vi "add_string_to_array_unique.vi"(8 "error in (no error)":errorcluster, 10 "strings to add":string[](array[string])=["subcomponent_cluster.ctl"], 11 "array in":string[](array[string])) -> (0 "error out":errorcluster, 3 "array out":string[](array[string]))   [LabVIEW 2010]
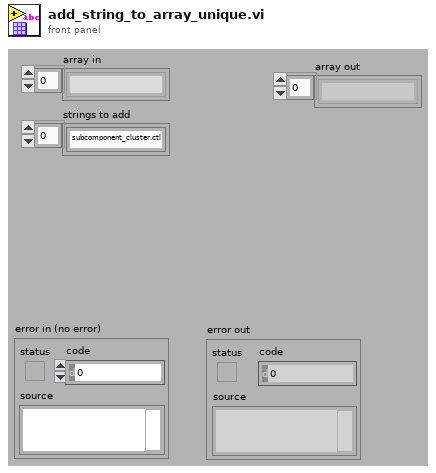
[diagram p1: front panel]
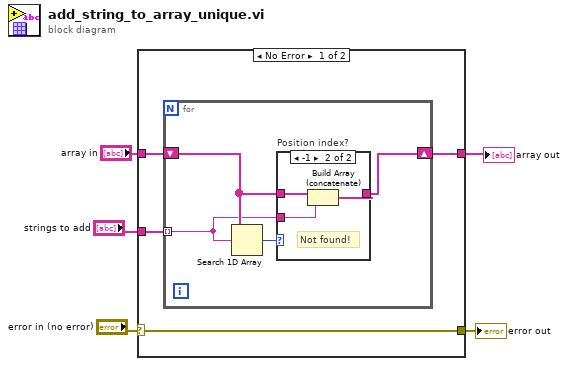
[diagram p0: block diagram]
diagram:
  n1 = case shown="No Error" "error in (no error)" {
    selector: "error in (no error)" -> [w7 w18]
    tunnel: [w9 w19] -> w5
    tunnel: "array in" -> [w8 w19]
    tunnel: [w7 w18] -> w2
    tunnel: "strings to add" -> [w6 _]
    frame No Error {
      n2 = for {
        tunnel: w6 -> [w10] mode=indexing
        shift-right: [w11] -> w9
        shift-left: w8 -> [w12]
        n3 = Search 1D Array(1D array=w12, element=w10) -> (index of element=w13:i32)  [unwired: 1 in]
        n4 = case "Position index?" shown="-1" w13 {
          tunnel: w12 -> [w14 w17]
          tunnel: w10 -> [_ w16]
          tunnel: [w14 w15] -> w11
          frame Default {
            # "Found!"
          }
          frame -1 {
            # "Not found!"
            n5 = Build Array (concatenate)(w17, w16) -> (w15:string[])
          }
        }
      }
    }
    frame Error {
    }
  }
  "array out" <- w5
  "error out" <- w2
